vi "initialise LEDs.vi"() -> (0 "error out":errorcluster {"code" format="%.0x"}, 3 "LED handle":refnum<visa-resource-name> caption="instrument handle out")   [LabVIEW 2017]
uses:
  <vilib>/Instr/_visa.llb/VISA Configure Serial Port (Instr).vi
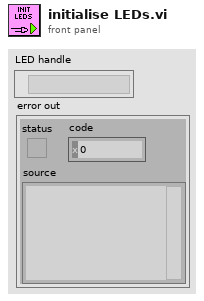
[diagram p1: front panel]
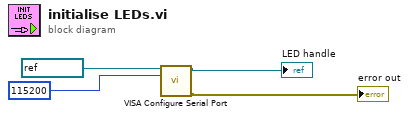
[diagram p0: block diagram]
diagram:
  n1 = call-poly "VISA Configure Serial Port"("VISA resource name"=refnum<visa-resource-name> "COM3", "baud rate (9600)"=u32 115200) -> ("VISA resource name out"=→"LED handle":refnum<visa-resource-name>, "error out"=→"error out":errorcluster)  [unwired: 12 in]
